vi "Create NI 9423 - Counter PWM Input.vi"(8 "error in":errorcluster, 10 "channel settings":T1[](array[typedef])) -> (0 "error out":errorcluster, 3 "module out":refnum<class "NI 9423.lvclass">)   [LabVIEW 2017, in "NI 9423.lvclass"]
uses:
  NI 9423.lvclass
  Mode Classes/Controls/counter pwm input channel settings.ctl
  Channel Classes/PWM Input Channel/Measurement Type.ctl
  Mode Classes/Counter PWM Input Mode/Counter PWM Input Mode.lvclass
  C:/dev/github.com/debryant/niveristand-scan-engine-ethercat-custom-device/Custom Device Source/Scripting/Modules/Mode Classes/Mode/Mode.lvclass
  b6df024b-8339-4a82-ba1a-1f387143499d.vi
  Channel Classes/PWM Input Channel/PWM Input Channel.lvclass
  Scan Engine Scripting.lvlib
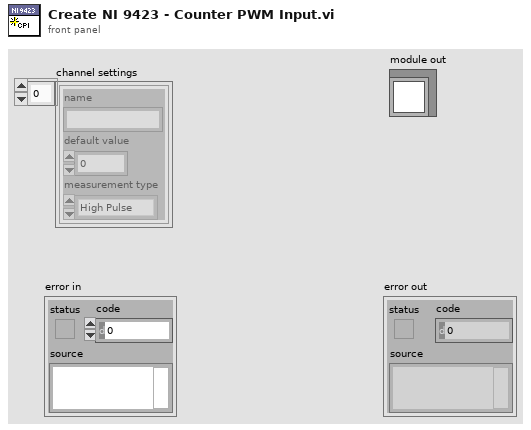
[diagram p1: front panel]
types:
  T1 = typedef "Scan Engine Scripting.lvlib/counter pwm input channel settings.ctl" = cluster{"name":string, "default value":dbl, "measurement type":T2}
  T2 = typedef "Scan Engine Scripting.lvlib/PWM Input Channel.lvclass/Measurement Type.ctl" = enum16{"High Pulse", "Low Pulse", "Most Recent"}
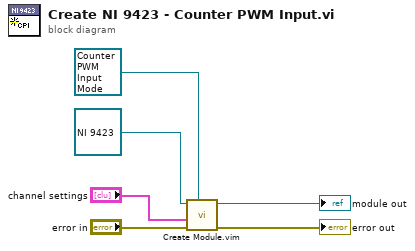
[diagram p0: block diagram]
diagram:
  n1 = call "Create Module.vim"("mode in"=refnum<class "Counter PWM Input Mode.lvclass"> refnum ("Scan Engine Scripting.lvlib:Counter PWM Input Mode.lvclass"), "error in"="error in", "channel settings"="channel settings", "module in"=refnum<class "NI 9423.lvclass"> refnum ("NI 9423.lvclass")) -> ("error out"=→"error out":errorcluster, "module out"=→"module out":refnum<class "NI 9423.lvclass">)  [unwired: 6 in]
